vi "Draw Ellipse (ARGB).vi"(4 "Ellipse Angles (Default: No rotation & full)":T2={"Rotation"=0.0, "Start"=0.0, "Stop"=360.0}, 5 "Thickness (Default: 1)":i32=1, 6 "OpenCV Line Type (Default LINE_8)":T6=enum."LINE_8", 7 "ARGB Colour":T5={"Alpha"=255, "RGB"=0}, 8 "error in (no error)":errorcluster, 9 "Axes":T1, 10 "Centre":T3, 11 "ARGB Image in":T4) -> (0 "error out":errorcluster, 3 "ARGB Image":T4)   [LabVIEW 2020, in "image.lvlib"]
doc: "Draw an elipse at the specified centre-point with the given Axes and Rotation."
uses:
  image.lvlib
  Line Type.ctl
  ARGB Image.ctl
  ARGB Colour.ctl
  common/Image Point (Integer).ctl
  Ellipse Angles.ctl
  common/Image Size (Integer).ctl
  eaaaec5c-60e1-4320-b5ad-f9d454208055.vi
  <vilib>/Utility/error.llb/Error Cluster From Error Code.vi
  common/common.lvlib
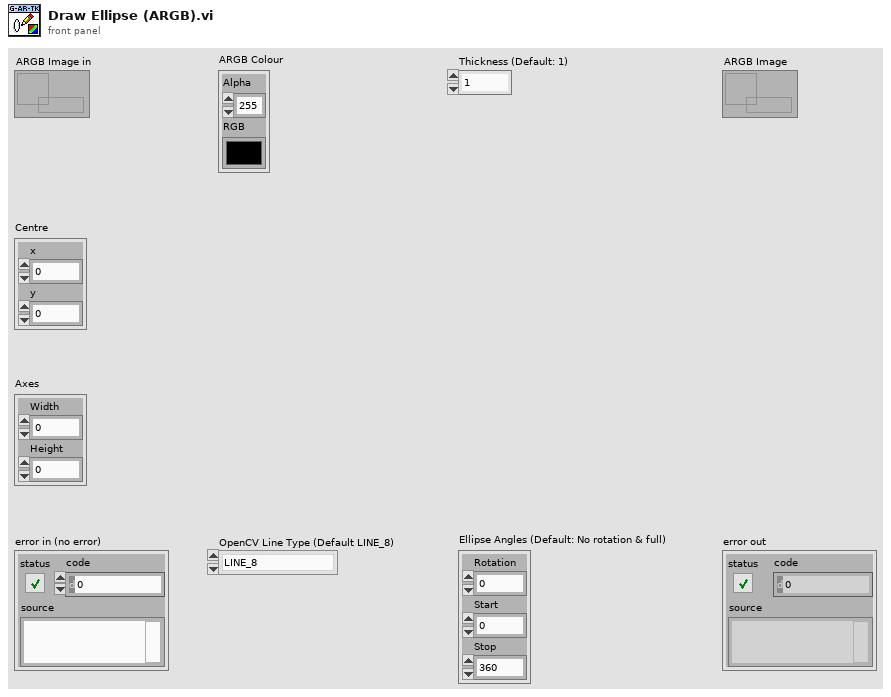
[diagram p1: front panel]
types:
  T1 = typedef "common.lvlib/Image Size (Integer).ctl" = cluster{"Width":u16, "Height":u16}
  T2 = typedef "image.lvlib/Ellipse Angles.ctl" = cluster{"Rotation":dbl, "Start":dbl, "Stop":dbl}
  T3 = typedef "common.lvlib/Image Point (Integer).ctl" = cluster{"x":i32, "y":i32}
  T4 = typedef "image.lvlib/ARGB Image.ctl" = refnum<data-value>
  T5 = typedef "image.lvlib/ARGB Colour.ctl" = cluster{"Alpha":u8, "RGB":u32}
  T6 = typedef "image.lvlib/Line Type.ctl" = enum8{"FILLED", "LINE_4", "LINE_8", "LINE_AA"}
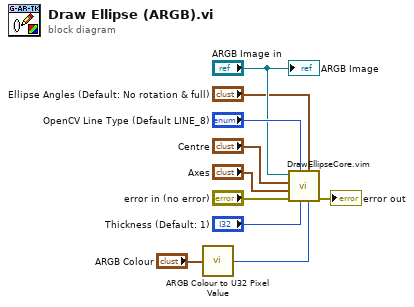
[diagram p0: block diagram]
diagram:
  n1 = call "ARGB Colour to U32 Pixel Value.vi"("ARGB Colour"="ARGB Colour") -> ("U32 Colour"=w5:u32)
  n2 = call "DrawEllipseCore.vim"("Colour"=w5, "Ellipse Angles"="Ellipse Angles (Default: No rotation & full)", "Thickness"="Thickness (Default: 1)", "OpenCV Line Type"="OpenCV Line Type (Default LINE_8)", "error in (no error)"="error in (no error)", "Axes"="Axes", "Centre"="Centre", "Src"="ARGB Image in") -> ("error out"=→"error out":errorcluster)  [unwired: 3 in]
  "ARGB Image" <- "ARGB Image in"
